vi "Draw.vi"(8 "error in (no error)":errorcluster, 10 "2D Picture in":picture, 11 "TriangleR in":refnum<class "TriangleL.lvclass">) -> (0 "error out":errorcluster, 2 "2D Picture out":picture, 3 "TriangleR out":refnum<class "TriangleL.lvclass">)   [LabVIEW 2021, in "Picture2D.lvlib" / "TriangleL.lvclass"]
uses:
  TriangleL.lvclass
  C:/Users/daal/OneDrive/LabVIEW/Class/Picture2D/Shape/Shape.lvclass
  C:/Users/daal/OneDrive/LabVIEW/Class/Picture2D/Triangle/Triangle.lvclass
  C:/Users/daal/OneDrive/LabVIEW/Class/Picture2D/Polygone/Polygone.lvclass
  Pen/Pen.lvclass
  Color/Color.lvclass
  Point/Point.lvclass
  TriangleL.lvclass/TriangleL.ctl
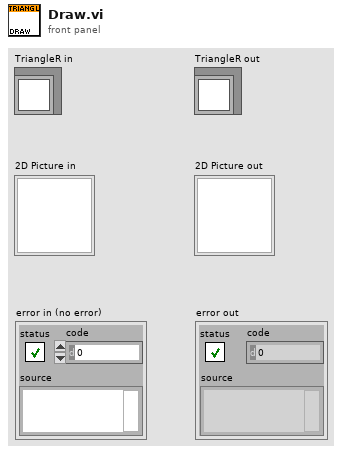
[diagram p1: front panel]
types:
  T1 = cluster{"Width":u16, "Style":enum32{"Solid", "Dash", "Dot", "DashDot", "DashDotDot"}}
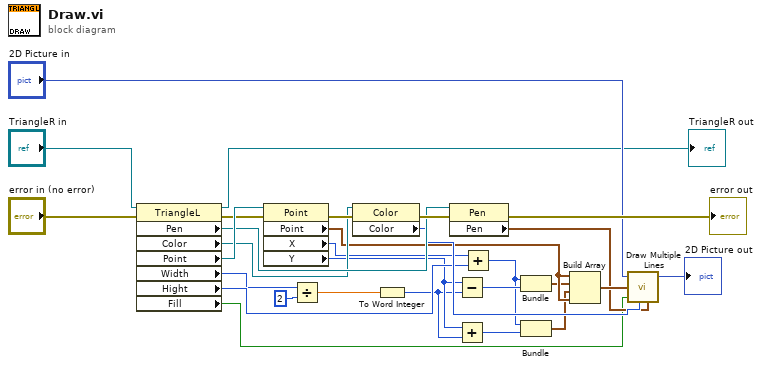
[diagram p0: block diagram]
diagram:
  n1 = property class="TriangleL"(reference="TriangleR in", error in="error in (no error)") -> (reference out=→"TriangleR out":refnum<class "TriangleL.lvclass">, error out=w28:errorcluster, "Pen"=w25:refnum<class "Pen.lvclass">, "Color"=w24:refnum<class "Color.lvclass">, "Point"=w29:refnum<class "Point.lvclass">, "Width"=w13:i16, "Hight"=w15:i16, "Fill"=w19:bool)
  n2 = property class="Point"(reference=w29, error in=w28) -> (error out=w27:errorcluster, "Point"=w22:cluster{"x":i16, "y":i16}, "X"=w16:i16, "Y"=w6:i16)  [unwired: 1 out]
  n3 = Divide(x=w13, y=i16 2) -> (x/y=w11:dbl)
  n4 = property class="Color"(reference=w24, error in=w27) -> (error out=w26:errorcluster, "Color"=w23:u32)  [unwired: 1 out]
  n5 = To Word Integer(number=w11) -> (16bit integer=w5:i16)
  n6 = property class="Pen"(reference=w25, error in=w26) -> (error out=→"error out":errorcluster, "Pen"=w20:T1)  [unwired: 1 out]
  n7 = Subtract(x=w6, y=w5) -> (x-y=w10:i16)
  n8 = Add(x=w6, y=w5) -> (x+y=w8:i16)
  n9 = Add(x=w16, y=w15) -> (x+y=w9:i16)
  n10 = Bundle(w9, w10) -> (w14:cluster{i16, i16})  [unwired: 1 in]
  n11 = Bundle(w9, w8) -> (w7:cluster{i16, i16})  [unwired: 1 in]
  n12 = Build Array(w22, w14, w7, w22) -> (w21:cluster{"x":i16, "y":i16}[])
  n13 = call <vilib>:"Draw Multiple Lines.vi"("picture"="2D Picture in", "line endpoints"=w21, "fill?(F)"=w19, "color(black)"=w23, "pen"=w20) -> ("new picture"=→"2D Picture out":picture)  [unwired: 4 in]
